vi "Get Offset and Span.vi"(7 "calbuffer":u8[](array[numeric]), 8 "error in (no error)":errorcluster, 10 "nScale":i32 min=0 max=8, 11 "nWhichChan":i32=1 min=1 max=4) -> (0 "error out":errorcluster, 1 "*pnChanSpanOffset":u16, 2 "*pnChanZeroOffset":u16)   [LabVIEW 2015]
panel:
  out "number 2":i32
  out "number":i32
  in  "calbuffer 3":u8[](array[numeric])=[3, 0, 86, 49, 50, 48, 48, 66, 70, 53, 70, 0, 0, 0, 64, 108, 233, 17, 0, 0, 0, 0, 48, 50, 45, 48, 54, 45, 50, 48, 49, 50, 79, 110, 67, 111, 114, 101, 0, 13, 1, 0, 0, 0, 64, 165, 233, 17, 64, 165, 233, 17, 69, 65, 80, 48, 50, 50, 54, 76, 53, 48, 0, 0, 160, 219, 233, 17, 152, 104, 38, 6, 56, 0, 0, 0, 48, 53, 45, 48, 51, 45, 50, 48, 49, 50, 83, 83, 80, 0, 232, 245, 243, 1, 225, 32, 248, 156, 1, 89, 190, 248, 8, 252, 203, 3, 1, 0, 0, 0, 255, 3, 255, 3, 0, 0, 0, 0, 0, 0, 64, 156, 0, 0, 0, 0, 0, 0, 64, 156, 0, 0, 0, 0, 0, 0, 64, 156, 0, 0, 0, 0, 0, 0, 64, 156, 0, 0, 0, 0, 0, 0, 64, 156, 0, 0, 0, 0, 0, 0, 64, 156, 0, 0, 0, 0, 0, 0, 64, 156, 0, 0, 0, 0, 0, 0, 64, 156, 0, 0, 0, 0, 0, 0, 64, 156, 0, 0, 0, 0, 0, 0, 64, 156, 0, 0, 0, 0, 0, 0, 0, 0, 0, 0, 0, 0, 0, 0, 0, 0, 0, 0, 0, 0, 0, 0, 0, 0, 0, 0, 0, 0, 0, 0, 0, 0, 0, 0, 0, 0, 0, 0, 0, 0, 0, 0, 186, 0, 255, 255, 3, 0, 255, 255, 3, 0, 255, 255, 3, 0, 255, 255, 3, 0, 238, 7, 34, 15, 248, 7, 32, 15, 1, 8, 63, 15, 2, 8, 53, 15, 3, 8, 44, 15, 255, 7, 155, 15, 1, 8, 148, 15, 3, 8, 142, 15, 5, 8, 182, 15, 254, 7, 54, 15, 8, 8, 45, 15, 15, 8, 80, 15, 17, 8, 71, 15, 18, 8, 55, 15, 14, 8, 177, 15, 16, 8, 170, 15, 17, 8, 158, 15, 19, 8, 194, 15, 0, 8, 44, 15, 13, 8, 39, 15, 23, 8, 82, 15, 24, 8, 74, 15, 26, 8, 56, 15, 22, 8, 186, 15, 24, 8, 181, 15, 25, 8, 167, 15, 26, 8, 207, 15, 35, 8, 141, 15, 36, 8, 124, 15, 33, 8, 150, 15, 33, 8, 138, 15, 32, 8, 119, 15, 32, 8, 188, 15, 32, 8, 179, 15, 32, 8, 163, 15, 31, 8, 182, 15, 0, 0, 0, 0, 85, 4, 0, 0, 0, 0, 0, 0, 6, 8, 38, 6, 19, 8, 228, 9, 2, 0, 255, 15, 102, 8, 47, 12, 36, 8, 207, 11, 33, 8, 209, 11, 32, 8, 212, 11, 32, 8, 211, 11, 32, 8, 215, 11, 0, 0, 0, 0, 0, 0, 0, 0, 0, 0, 0, 0, 0, 0, 0, 0, 0, 0, 0, 0, 0, 0, 0, 0, 0, 0, 0, 0, 0, 0, 0, 0, 0, 0, 0, 0, 0, 0, 0, 0, 0, 0, 0, 0, 0, 0, 0, 0, 0, 0, 0, 0, 0, 0, 0, 0, 0, 0, 0, 0, 0, 0, 0, 0, 0, 0, 0, 0, 0, 0, 0, 0, 24, 84, 0, 0, 0, 0, 0, 0, 0, 0, 0, 0, 0, 0, 0, 0, 0, 0, 0, 0, 0, 0, 0, 0, 0, 0, 0, 0, 0, 0, 0, 0, 0, 0, 0, 0, 0, 0, 0, 0, 0, 0, 0, 0, 0, 0, 0, 0, 0, 0, 0, 0, 0, 0, 0, 0, 0, 0, 0, 0, 0, 0, 0, 0, 0, 0, 0, 0, 0, 0, 0, 0, 0, 0, 0, 0, 0, 0, 0, 0, 0, 0, 0]
  in  "all of the appendix":string="3\tAPPENDIX1 - CALIBRATION DATA STRUCTURE\nThe EEPROM is used to store Factory calibration data, Scope Serial number and other useful information. The format of the memory is listed in the table below:\nEerom size = 4kBytes\nInitialization:\n1.\tclear all locations to 00h\n2.\twrite 16bit checksum at last 2 locations\n3.\tserial number and other things write only if calibration passes.\nInteger\t\tLeast significant Byte first\nShort\t\tLeast significant Byte first\nLong\t\tLeast significant Byte first\nString\t\tno null termination\n\nDescription\tFormat\tBytes\tLocation\nRevision of Eeprom format\tShort\t2\tBASE\nSerial number \tString\t20\tBASE+2\nDate of Manufacture (First time calibrated)\tString\t10\tBASE+22 \nLocation of Manufacture\tString\t20\tBASE+32 \nPrinted Circuit Board Assembly #\tString\t20\tBASE+52\nPrinted Circuit board Revision\tString\t2\tBASE+72\nNumber of Calibrations done\tInteger\t2\tBASE+74\nDate of Last Calibration\tString\t10\tBASE+76 \nLocation of Calibration\tString\t20\tBASE+86\nMaster Calibration Flag\tBOOL\t4\tBASE+106\nDCV_CALFLAGS Structure\tInteger\t2\tBASE+110 \nACV_CALFLAGS Structure\tInteger\t2\tBASE+112\nOHM_CALFLAGS Structure\tInteger\t2\tBASE+114\nMmDcVoltsCal structure (not used in Tripoli)\tInteger\t40\tBASE+116\nMmAcVoltsCal structure (not used in Tripoli)\tInteger\t40\tBASE+156\nOHM400Z - Zero error of the Ohms channel, 400 Ohm scale.\tInteger\t4\tBASE+196\nOHM400G - Gain for Ohms channel, 400 Ohm scale.\tInteger\t4\tBASE+200\nOHM4KZ - Zero error of the Ohms channel, 4 k Ohm scale.\tInteger\t4\tBASE+204\nOHM4KG - Gain for Ohms channel, 4 k Ohm scale.\tInteger\t4\tBASE+208\nOHM40KZ - Zero error of the Ohms channel, 40 k Ohm scale.\tInteger\t4\tBASE+212\nOHM40KG - Gain for Ohms channel, 40 k Ohm scale.\tInteger\t4\tBASE+216\nOHM400KZ - Zero error of the Ohms channel, 400 k Ohm scale.\tInteger\t4\tBASE+220\nOHM400KG - Gain for Ohms channel, 400 k Ohm scale.\tInteger\t4\tBASE+224\nOHM4MZ - Zero error of the Ohms channel, 4 M Ohm scale.\tInteger\t4\tBASE+228\nOHM4MG - Gain for Ohms channel, 4 M Ohm scale.\tInteger\t4\tBASE+232\nDPOT Setting\tShort\t2\tBASE+236\nChannel 1 CHAN_CALFLAGS Structure\tInteger\t4\tBASE+238\nChannel 2 CHAN_CALFLAGS Structure\tInteger\t4\tBASE+242\nChannel 3 CHAN_CALFLAGS Structure\tInteger\t4\tBASE+246\nChannel 4 CHAN_CALFLAGS Structure\tInteger\t4\tBASE+250\nCH1_1Z - Zero error channel 1, 1 Volt scale\tShort\t2\tBASE+254\nCH1_1G - Gain for channel 1, 1 volt scale\tShort\t2\tBASE+256\nCH2_1Z - Zero error channel 2, 1 Volt scale\tShort\t2\tBASE+258\nCH2_1G - Gain for channel 2, 1 volt scale\tShort\t2\tBASE+260\nCH3_1Z - Zero error channel 3, 1 Volt scale\tShort\t2\tBASE+262\nCH3_1G - Gain for channel 3, 1 volt scale\tShort\t2\tBASE+264\nCH4_1Z - Zero error channel 4, 1 Volt scale\tShort\t2\tBASE+266\nCH4_1G - Gain for channel 4, 1 volt scale\tShort\t2\tBASE+268\nCH1_2Z - Zero error channel 1, 2 Volt scale\tShort\t2\tBASE+270\nCH1_2G - Gain for channel 1, 2 volt scale\tShort\t2\tBASE+272\nCH2_2Z - Zero error channel 2, 2 Volt scale\tShort\t2\tBASE+274\nCH2_2G - Gain for channel 2, 2 volt scale\tShort\t2\tBASE+276\nCH3_2Z - Zero error channel 3, 2 Volt scale\tShort\t2\tBASE+278\nCH3_2G - Gain for channel 3, 2 volt scale\tShort\t2\tBASE+280\nCH4_2Z - Zero error channel 4, 2 Volt scale\tShort\t2\tBASE+282\nCH4_2G - Gain for channel 4, 2 volt scale\tShort\t2\tBASE+284\nCH1_5Z - Zero error channel 1, 5 Volt scale\tShort\t2\tBASE+286\nCH1_5G - Gain for channel 1, 5 volt scale\tShort\t2\tBASE+288\nCH2_5Z - Zero error channel 2, 5 Volt scale\tShort\t2\tBASE+290\nCH2_5G - Gain for channel 2, 5 volt scale\tShort\t2\tBASE+292\nCH3_5Z - Zero error channel 3, 5 Volt scale\tShort\t2\tBASE+294\nCH3_5G - Gain for channel 3, 5 volt scale\tShort\t2\tBASE+296\nCH4_5Z - Zero error channel 4, 5 Volt scale\tShort\t2\tBASE+298\nCH4_5G - Gain for channel 4, 5 volt scale\tShort\t2\tBASE+300\nCH1_10Z - Zero error channel 1, 10 Volt scale\tShort\t2\tBASE+302\nCH1_10G - Gain for channel 1, 10 volt scale\tShort\t2\tBASE+304\nCH2_10Z - Zero error channel 2, 10 Volt scale\tShort\t2\tBASE+306\nCH2_10G - Gain for channel 2, 10 volt scale\tShort\t2\tBASE+308\nCH3_10Z - Zero error channel 3, 10 Volt scale\tShort\t2\tBASE+310\nCH3_10G - Gain for channel 3, 10 volt scale\tShort\t2\tBASE+312\nCH4_10Z - Zero error channel 4, 10 Volt scale\tShort\t2\tBASE+314\nCH4_10G - Gain for channel 4, 10 volt scale\tShort\t2\tBASE+316\nCH1_20Z - Zero error channel 1, 20 Volt scale\tShort\t2\tBASE+318\nCH1_20G - Gain for channel 1, 20 volt scale\tShort\t2\tBASE+320\nCH2_20Z - Zero error channel 2, 20 Volt scale\tShort\t2\tBASE+322\nCH2_20G - Gain for channel 2, 20 volt scale\tShort\t2\tBASE+324\nCH3_20Z - Zero error channel 3, 20 Volt scale\tShort\t2\tBASE+326\nCH3_20G - Gain for channel 3, 20 volt scale\tShort\t2\tBASE+328\nCH4_20Z - Zero error channel 4, 20 Volt scale\tShort\t2\tBASE+330\nCH4_20G - Gain for channel 4, 20 volt scale\tShort\t2\tBASE+332\nCH1_50Z - Zero error channel 1, 50 Volt scale\tShort\t2\tBASE+334\nCH1_50G - Gain for channel 1, 50 volt scale\tShort\t2\tBASE+336\nCH2_50Z - Zero error channel 2, 50 Volt scale\tShort\t2\tBASE+338\nCH2_50G - Gain for channel 2, 50 volt scale\tShort\t2\tBASE+340\nCH3_50Z - Zero error channel 3, 50 Volt scale\tShort\t2\tBASE+342\nCH3_50G - Gain for channel 3, 50 volt scale\tShort\t2\tBASE+344\nCH4_50Z - Zero error channel 4, 50 Volt scale\tShort\t2\tBASE+346\nCH4_50G - Gain for channel 4, 50 volt scale\tShort\t2\tBASE+348\nCH1_100Z - Zero error channel 1, 100 Volt scale\tShort\t2\tBASE+350\nCH1_100G - Gain for channel 1, 100 volt scale\tShort\t2\tBASE+352\nCH2_100Z - Zero error channel 2, 100 Volt scale\tShort\t2\tBASE+354\nCH2_100G - Gain for channel 2, 100 volt scale\tShort\t2\tBASE+356\nCH3_100Z - Zero error channel 3, 100 Volt scale\tShort\t2\tBASE+358\nCH3_100G - Gain for channel 3, 100 volt scale\tShort\t2\tBASE+360\nCH4_100Z - Zero error channel 4, 100 Volt scale\tShort\t2\tBASE+362\nCH4_100G - Gain for channel 4, 100 volt scale\tShort\t2\tBASE+364\nCH1_200Z - Zero error channel 1, 200 Volt scale\tShort\t2\tBASE+366\nCH1_200G - Gain for channel 1, 200 volt scale\tShort\t2\tBASE+368\nCH2_200Z - Zero error channel 2, 200 Volt scale\tShort\t2\tBASE+370\nCH2_200G - Gain for channel 2, 200 volt scale\tShort\t2\tBASE+372\nCH3_200Z - Zero error channel 3, 200 Volt scale\tShort\t2\tBASE+374\nCH3_200G - Gain for channel 3, 200 volt scale\tShort\t2\tBASE+376\nCH4_200Z - Zero error channel 4, 200 Volt scale\tShort\t2\tBASE+378\nCH4_200G - Gain for channel 4, 200 volt scale\tShort\t2\tBASE+380\nCH1_400Z - Zero error channel 1, 400 Volt scale\tShort\t2\tBASE+382\nCH1_400G - Gain for channel 1, 400 volt scale\tShort\t2\tBASE+384\nCH2_400Z - Zero error channel 2, 400 Volt scale\tShort\t2\tBASE+386\nCH2_400G - Gain for channel 2, 400 volt scale\tShort\t2\tBASE+388\nCH3_400Z - Zero error channel 3, 400 Volt scale\tShort\t2\tBASE+390\nCH3_400G - Gain for channel 3, 400 volt scale\tShort\t2\tBASE+392\nCH4_400Z - Zero error channel 4, 400 Volt scale\tShort\t2\tBASE+394\nCH4_400G - Gain for channel 4, 400 volt scale\tShort\t2\tBASE+396\nAUXPSCALSTAT - Aux. PS Calibration Status\tBOOL\t4\tBASE+398\nAUXPSZ - Aux. PS Zero Error\tInteger\t4\tBASE+402\nAUXPSG - Gain for Aux. PS\tInteger\t4\tBASE+406\nPKSTR_CH1_10Z - Peak Stretch Zero error channel 1\tShort\t2\tBASE+410\nPKSTR_CH1_10G - Peak Stretch Gain for channel 1\tShort\t2\tBASE+412\nPKSTR_CH2_10Z - Peak Stretch Zero error channel 2\tShort\t2\tBASE+414\nPKSTR_CH2_10G - Peak Stretch Gain for channel 2\tShort\t2\tBASE+416\nPLATFORMTYPE - flag indicating if M4\tShort\t2\tBASE+418\nM4OHM_CALFLAGS Structure\tInteger\t2\tBASE+420\nM4_OHM50Z - Zero error of the M4 Ohms channel, 50 Ohm scale.\tShort\t2\tBASE+422\nM4_OHM50G - Gain for the M4 Ohms channel, 50 Ohm scale.\tShort\t2\tBASE+424\nM4_OHM1KZ - Zero error of the M4 Ohms channel, 1K Ohm scale.\tShort\t2\tBASE+426\nM4_OHM1KG - Gain for the M4 Ohms channel, 1K Ohm scale.\tShort\t2\tBASE+428\nM4_OHM10KZ - Zero error of the M4 Ohms channel, 10K Ohm scale.\tShort\t2\tBASE+430\nM4_OHM10KG - Gain for the M4 Ohms channel, 10K Ohm scale.\tShort\t2\tBASE+432\nM4_OHM100KZ - Zero error of the M4 Ohms channel, 100K Ohm scale.\tShort\t2\tBASE+434\nM4_OHM100KG - Gain for the M4 Ohms channel, 100 K Ohm scale.\tShort\t2\tBASE+436\nM4_OHM1MZ - Zero error of the M4 Ohms channel, 1M Ohm scale.\tShort\t2\tBASE+438\nM4_OHM1MG - Gain for the M4 Ohms channel, 1M Ohm scale.\tShort\t2\tBASE+440\nM4_OHM10MZ - Zero error of the M4 Ohms channel, 10M Ohm scale.\tShort\t2\tBASE+442\nM4_OHM10MG - Gain for the M4 Ohms channel, 10 M Ohm scale.\tShort\t2\tBASE+440\nPadding (72) reduced as items are added to this struct\tchar\t72\tBASE+442 (0x1BA)\n\t\t\t\nChecksum\tInteger\t2\tBASE+518 (0x14A)\n"
  in  "String":string="CH1_1Z - Zero error channel 1, 1 Volt scale\tShort\t2\tBASE+254\nCH1_1G - Gain for channel 1, 1 volt scale\tShort\t2\tBASE+256\nCH2_1Z - Zero error channel 2, 1 Volt scale\tShort\t2\tBASE+258\nCH2_1G - Gain for channel 2, 1 volt scale\tShort\t2\tBASE+260\nCH3_1Z - Zero error channel 3, 1 Volt scale\tShort\t2\tBASE+262\nCH3_1G - Gain for channel 3, 1 volt scale\tShort\t2\tBASE+264\nCH4_1Z - Zero error channel 4, 1 Volt scale\tShort\t2\tBASE+266\nCH4_1G - Gain for channel 4, 1 volt scale\tShort\t2\tBASE+268\nCH1_2Z - Zero error channel 1, 2 Volt scale\tShort\t2\tBASE+270\nCH1_2G - Gain for channel 1, 2 volt scale\tShort\t2\tBASE+272\nCH2_2Z - Zero error channel 2, 2 Volt scale\tShort\t2\tBASE+274\nCH2_2G - Gain for channel 2, 2 volt scale\tShort\t2\tBASE+276\nCH3_2Z - Zero error channel 3, 2 Volt scale\tShort\t2\tBASE+278\nCH3_2G - Gain for channel 3, 2 volt scale\tShort\t2\tBASE+280\nCH4_2Z - Zero error channel 4, 2 Volt scale\tShort\t2\tBASE+282\nCH4_2G - Gain for channel 4, 2 volt scale\tShort\t2\tBASE+284\nCH1_5Z - Zero error channel 1, 5 Volt scale\tShort\t2\tBASE+286\nCH1_5G - Gain for channel 1, 5 volt scale\tShort\t2\tBASE+288\nCH2_5Z - Zero error channel 2, 5 Volt scale\tShort\t2\tBASE+290\nCH2_5G - Gain for channel 2, 5 volt scale\tShort\t2\tBASE+292\nCH3_5Z - Zero error channel 3, 5 Volt scale\tShort\t2\tBASE+294\nCH3_5G - Gain for channel 3, 5 volt scale\tShort\t2\tBASE+296\nCH4_5Z - Zero error channel 4, 5 Volt scale\tShort\t2\tBASE+298\nCH4_5G - Gain for channel 4, 5 volt scale\tShort\t2\tBASE+300\nCH1_10Z - Zero error channel 1, 10 Volt scale\tShort\t2\tBASE+302\nCH1_10G - Gain for channel 1, 10 volt scale\tShort\t2\tBASE+304\nCH2_10Z - Zero error channel 2, 10 Volt scale\tShort\t2\tBASE+306\nCH2_10G - Gain for channel 2, 10 volt scale\tShort\t2\tBASE+308\nCH3_10Z - Zero error channel 3, 10 Volt scale\tShort\t2\tBASE+310\nCH3_10G - Gain for channel 3, 10 volt scale\tShort\t2\tBASE+312\nCH4_10Z - Zero error channel 4, 10 Volt scale\tShort\t2\tBASE+314\nCH4_10G - Gain for channel 4, 10 volt scale\tShort\t2\tBASE+316\nCH1_20Z - Zero error channel 1, 20 Volt scale\tShort\t2\tBASE+318\nCH1_20G - Gain for channel 1, 20 volt scale\tShort\t2\tBASE+320\nCH2_20Z - Zero error channel 2, 20 Volt scale\tShort\t2\tBASE+322\nCH2_20G - Gain for channel 2, 20 volt scale\tShort\t2\tBASE+324\nCH3_20Z - Zero error channel 3, 20 Volt scale\tShort\t2\tBASE+326\nCH3_20G - Gain for channel 3, 20 volt scale\tShort\t2\tBASE+328\nCH4_20Z - Zero error channel 4, 20 Volt scale\tShort\t2\tBASE+330\nCH4_20G - Gain for channel 4, 20 volt scale\tShort\t2\tBASE+332\nCH1_50Z - Zero error channel 1, 50 Volt scale\tShort\t2\tBASE+334\nCH1_50G - Gain for channel 1, 50 volt scale\tShort\t2\tBASE+336\nCH2_50Z - Zero error channel 2, 50 Volt scale\tShort\t2\tBASE+338\nCH2_50G - Gain for channel 2, 50 volt scale\tShort\t2\tBASE+340\nCH3_50Z - Zero error channel 3, 50 Volt scale\tShort\t2\tBASE+342\nCH3_50G - Gain for channel 3, 50 volt scale\tShort\t2\tBASE+344\nCH4_50Z - Zero error channel 4, 50 Volt scale\tShort\t2\tBASE+346\nCH4_50G - Gain for channel 4, 50 volt scale\tShort\t2\tBASE+348\nCH1_100Z - Zero error channel 1, 100 Volt scale\tShort\t2\tBASE+350\nCH1_100G - Gain for channel 1, 100 volt scale\tShort\t2\tBASE+352\nCH2_100Z - Zero error channel 2, 100 Volt scale\tShort\t2\tBASE+354\nCH2_100G - Gain for channel 2, 100 volt scale\tShort\t2\tBASE+356\nCH3_100Z - Zero error channel 3, 100 Volt scale\tShort\t2\tBASE+358\nCH3_100G - Gain for channel 3, 100 volt scale\tShort\t2\tBASE+360\nCH4_100Z - Zero error channel 4, 100 Volt scale\tShort\t2\tBASE+362\nCH4_100G - Gain for channel 4, 100 volt scale\tShort\t2\tBASE+364\nCH1_200Z - Zero error channel 1, 200 Volt scale\tShort\t2\tBASE+366\nCH1_200G - Gain for channel 1, 200 volt scale\tShort\t2\tBASE+368\nCH2_200Z - Zero error channel 2, 200 Volt scale\tShort\t2\tBASE+370\nCH2_200G - Gain for channel 2, 200 volt scale\tShort\t2\tBASE+372\nCH3_200Z - Zero error channel 3, 200 Volt scale\tShort\t2\tBASE+374\nCH3_200G - Gain for channel 3, 200 volt scale\tShort\t2\tBASE+376\nCH4_200Z - Zero error channel 4, 200 Volt scale\tShort\t2\tBASE+378\nCH4_200G - Gain for channel 4, 200 volt scale\tShort\t2\tBASE+380\nCH1_400Z - Zero error channel 1, 400 Volt scale\tShort\t2\tBASE+382\nCH1_400G - Gain for channel 1, 400 volt scale\tShort\t2\tBASE+384\nCH2_400Z - Zero error channel 2, 400 Volt scale\tShort\t2\tBASE+386\nCH2_400G - Gain for channel 2, 400 volt scale\tShort\t2\tBASE+388\nCH3_400Z - Zero error channel 3, 400 Volt scale\tShort\t2\tBASE+390\nCH3_400G - Gain for channel 3, 400 volt scale\tShort\t2\tBASE+392\nCH4_400Z - Zero error channel 4, 400 Volt scale\tShort\t2\tBASE+394\nCH4_400G - Gain for channel 4, 400 volt scale\tShort\t2\tBASE+396\nAUXPSCALSTAT - Aux. PS Calibration Status\tBOOL\t4\tBASE+398\nAUXPSZ - Aux. PS Zero Error\tInteger\t4\tBASE+402\nAUXPSG - Gain for Aux. PS\tInteger\t4\tBASE+406"
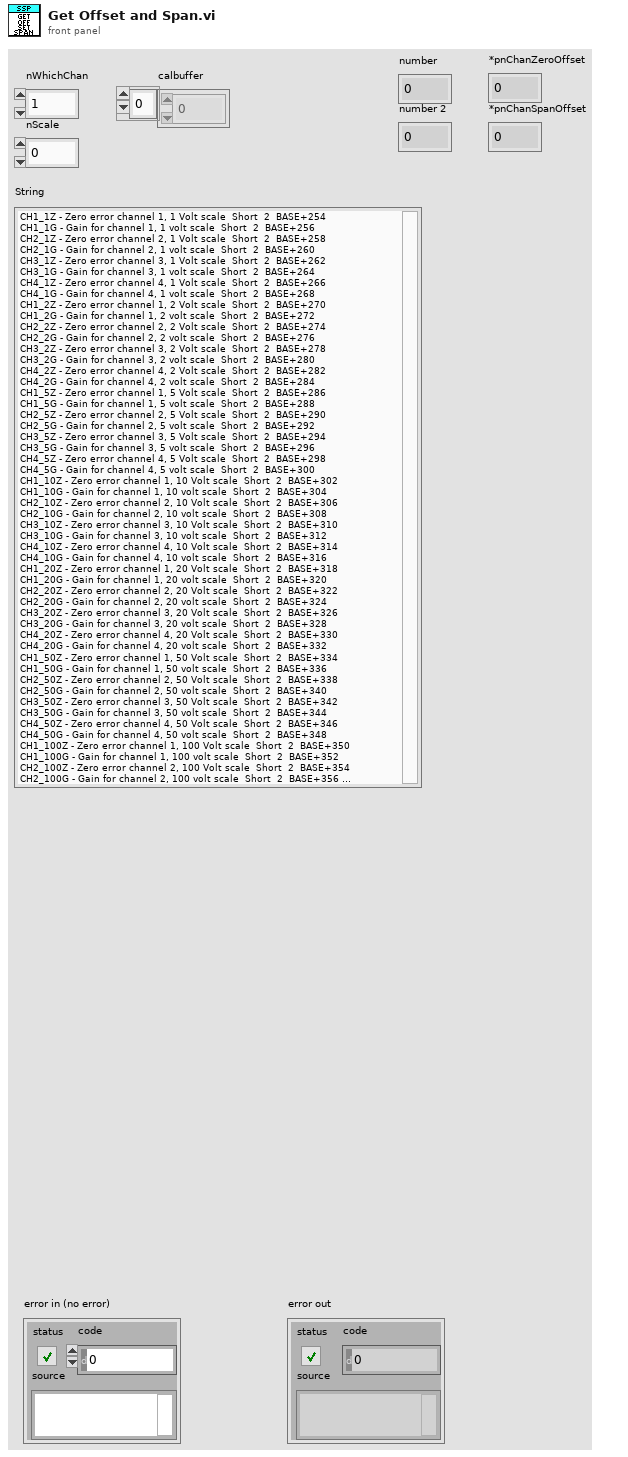
[diagram p1: front panel]
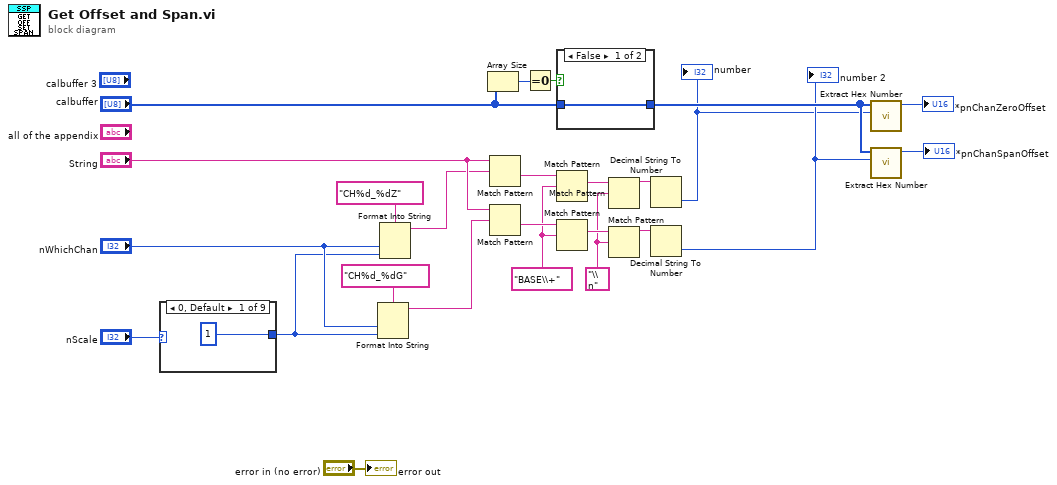
[diagram p0: block diagram]
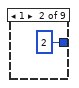
[diagram p2: hidden frame]
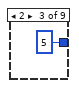
[diagram p3: hidden frame]
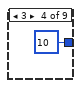
[diagram p4: hidden frame]
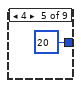
[diagram p5: hidden frame]
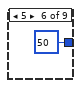
[diagram p6: hidden frame]
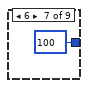
[diagram p7: hidden frame]
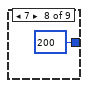
[diagram p8: hidden frame]
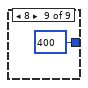
[diagram p9: hidden frame]
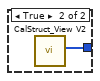
[diagram p10: hidden frame]
diagram:
  w2 = "\\n"
  w3 = "BASE\\+" ("regular expression")
  n1 = case shown="0, Default" "nScale" {
    tunnel: [1 2 5 10 20 50 100 200 400] -> w4
    frame 0, Default {
    }
    frame 1 {
    }
    frame 2 {
    }
    frame 3 {
    }
    frame 4 {
    }
    frame 5 {
    }
    frame 6 {
    }
    frame 7 {
    }
    frame 8 {
    }
  }
  n2 = Format Into String(format string="CH%d_%dG", "nWhichChan", w4) -> (resulting string=w7:string)  [unwired: 2 in, 1 out]
  n3 = Format Into String(format string="CH%d_%dZ", "nWhichChan", w4) -> (resulting string=w8:string)  [unwired: 2 in, 1 out]
  n4 = Array Size(array="calbuffer") -> (size(s)=w24:i32)
  n5 = Match Pattern(string="String", regular expression=w8) -> (after substring=w13:string)  [unwired: 1 in, 3 out]
  n6 = Match Pattern(string="String", regular expression=w7) -> (after substring=w9:string)  [unwired: 1 in, 3 out]
  n7 = Equal To 0?(x=w24) -> (x = 0?=w23:bool)
  n8 = case shown="False" w23 {
    tunnel: [w35 w36] -> w21
    tunnel: "calbuffer" -> [w35 _]
    frame False {
    }
    frame True {
      n9 = call "CalStruct_View V2.vi"() -> ("calbuffer"=w36:u8[])  [unwired: 9 in, 2 out]
    }
  }
  n10 = Match Pattern(string=w13, regular expression=w3) -> (after substring=w18:string)  [unwired: 1 in, 3 out]
  n11 = Match Pattern(string=w9, regular expression=w3) -> (after substring=w11:string)  [unwired: 1 in, 3 out]
  n12 = Match Pattern(string=w18, regular expression=w2) -> (before substring=w17:string)  [unwired: 1 in, 3 out]
  n13 = Match Pattern(string=w11, regular expression=w2) -> (before substring=w12:string)  [unwired: 1 in, 3 out]
  n14 = Decimal String To Number(string=w17) -> (number=w1:i32)  [unwired: 2 in, 1 out]
  "number" <- w1
  n15 = Decimal String To Number(string=w12) -> (number=w6:i32)  [unwired: 2 in, 1 out]
  "number 2" <- w6
  n16 = call "Extract Hex Number.vi"("index"=w1, "unsigned byte array"=w21) -> ("Numeric"=→"*pnChanZeroOffset":u16)  [unwired: 9 in]
  n17 = call "Extract Hex Number.vi"("index"=w6, "unsigned byte array"=w21) -> ("Numeric"=→"*pnChanSpanOffset":u16)  [unwired: 9 in]
  "error out" <- "error in (no error)"
